vi "Dequeue Message.vi"(8 "error in":errorcluster, 11 "message queue":refnum<queue>) -> (0 "error out":errorcluster, 1 "Message Data":variant, 2 "Message":string, 3 "dup message queue":refnum<queue>)   [LabVIEW 2024, in "DSA_CFG_ACQ.lvlib" / "SFPMessage Queue.lvlib"]
doc: "This VI pulls messages off the Message Queue. It has special error handling to account for an error occurring on the last iteration of the Message Handling Loop.\n\nNo Error - normal Dequeue Element operation.\nError - check if it is an error code we wish to ignore. If so, clear the error and perform a normal Dequeue Element. If not, output the error, and put a 'Stop' message on the Message Queue."
uses:
  SFPMessage Queue.lvlib
  Message Cluster.ctl
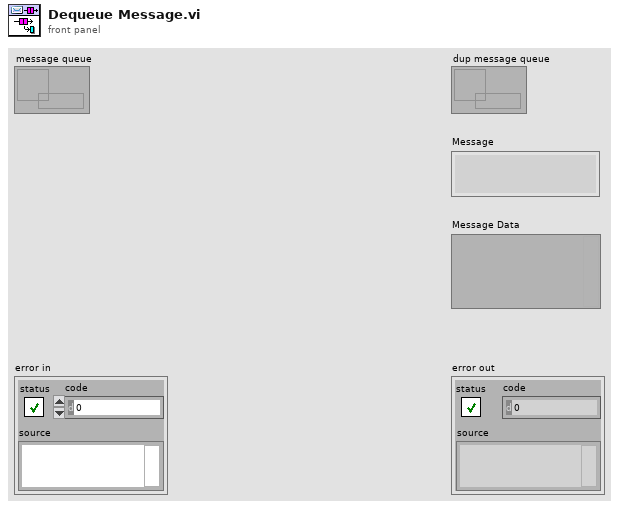
[diagram p1: front panel]
types:
  T1 = typedef "DSA_CFG_ACQ.lvlib/SFPMessage Queue.lvlib/Message Cluster.ctl" = cluster{"Message":string, "Message Data":variant}
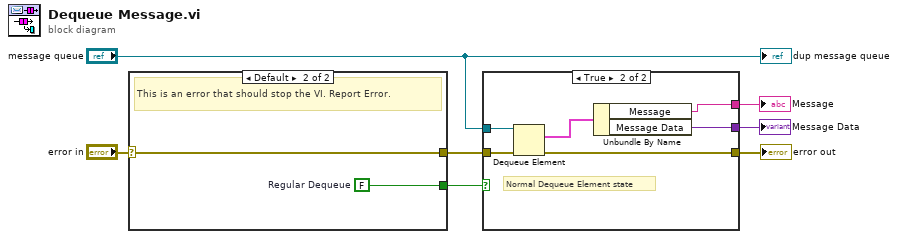
[diagram p0: block diagram]
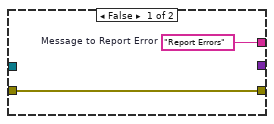
[diagram p2: hidden frame]
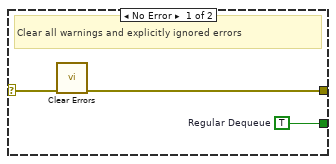
[diagram p3: hidden frame]
diagram:
  n1 = case shown="Default" "error in" {
    selector: "error in" -> [w9 w12]
    tunnel: [w8 w12] -> w5
    tunnel: [w10 w11] -> w4
    frame No Error {
      w10 = TRUE  # Regular Dequeue
      # "Clear all warnings and explicitly ignored errors"
      n2 = call <vilib>:"Clear Errors.vi"("error in (no error)"=w9) -> ("error out"=w8:errorcluster)  [unwired: 5 in, 1 out]
    }
    frame Default {
      w11 = FALSE  # Regular Dequeue
      # "This is an error that should stop the VI. Report Error."
    }
  }
  n3 = case shown="True" w4 {
    tunnel: [w14 w20] -> w6
    tunnel: w5 -> [w14 w19]
    tunnel: "message queue" -> [_ w18]
    tunnel: [w13 w16] -> w3
    tunnel: [_ w15] -> w2
    frame False {
      w13 = "Report Errors"  # Message to Report Error
    }
    frame True {
      # "Normal Dequeue Element state"
      n4 = Dequeue Element(queue=w18, error in (no error)=w19) -> (element=w17:T1, error out=w20:errorcluster)  [unwired: 1 in, 2 out]
      n5 = Unbundle By Name(w17) -> ("Message"=w16:string, "Message Data"=w15:variant)
    }
  }
  "error out" <- w6
  "Message" <- w3
  "Message Data" <- w2
  "dup message queue" <- "message queue"
